vi "Modulized Autonomous Block.vi"(9 "Power":dbl format="%#_13g", 10 "run time in seconds":dbl, 11 "Direction":dbl) -> (3 "Output":T1 {"Direction" format="%#_13g"; "Rotation(Angle)" format="%#_13g"})   [LabVIEW 2014]
uses:
  Support Code/Robot Global Data.vi
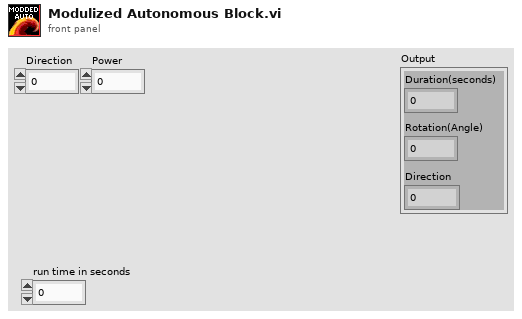
[diagram p1: front panel]
types:
  T1 = cluster{"Duration(seconds)":i32, "Rotation(Angle)":dbl, "Direction":dbl}
  T2 = cluster{"Speed":dbl, "Direction":dbl, "Rotation":dbl}
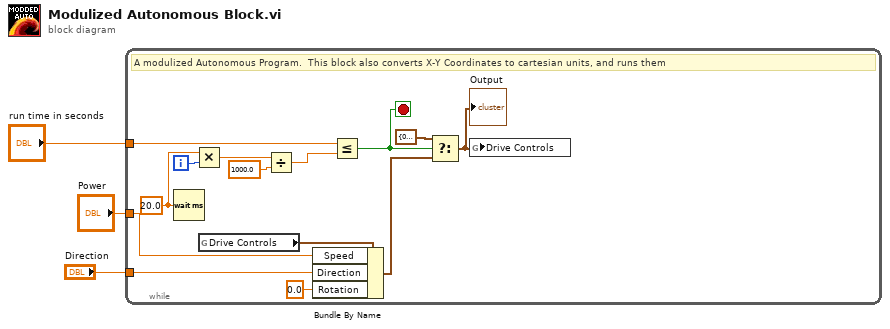
[diagram p0: block diagram]
diagram:
  n1 = while {
    tunnel: "Power" -> [w17]
    tunnel: "run time in seconds" -> [w11]
    tunnel: "Direction" -> [w7]
    i -> [w13]
    stop <- w6 stop-if-true
    w12 = 20.0 ("milliseconds to wait")
    # "A modulized Autonomous Program.  This block also converts X-Y Coordinates to cartesian units, and runs them"
    n2 = Wait (ms)(milliseconds to wait=w12) -> ()  [unwired: 1 out]
    n3 = Multiply(x=w12, y=w13) -> (x*y=w9:dbl)
    n4 = global read "Robot Global Data.vi" "Drive Controls"() -> (w5:T2)
    n5 = Divide(x=w9, y=1000.0) -> (x/y=w8:dbl)
    n6 = Bundle By Name(cluster=w5, "Speed"=w17, "Direction"=w7, "Rotation"=0.0) -> (w14:T2)
    n7 = Less Or Equal?(x=w11, y=w8) -> (x <= y?=w6:bool)
    n8 = Select(t=T2 {"Speed"=0.0, "Direction"=0.0, "Rotation"=0.0}, s=w6, f=w14) -> (s? t:f=w16:T2)
    "Output" <- w16
    n9 = global write "Robot Global Data.vi" "Drive Controls"(w16) -> ()
  }
